vi "DSF.Engine.BuilderManager.Initialize Builders.vi"(7 "Framework Cache":refnum<class "DSF.Engine.Memory.Cache.Framework.lvclass">, 8 "error in (no error)":errorcluster, 10 "Builder Statuses":refnum<class "Status.Builder.lvclass">[](array[class]), 11 "Builder Manager in":refnum<class "DSF.Engine.BuilderManager.lvclass">) -> (0 "error out":errorcluster, 3 "Builder Manager out":refnum<class "DSF.Engine.BuilderManager.lvclass">)   [LabVIEW 2016, in "DSF.Engine.lvlib" / "DSF.Engine.BuilderManager.lvclass"]
uses:
  DSF.Engine.BuilderManager.lvclass
  Cache/DSF.Engine.Memory.Cache.Framework.lvclass
  Status/Status.Builder.lvclass
  DSF.Engine.BuilderManager.lvclass/DSF.Engine.BuilderManager.ctl
  Builder/DSF.Engine.Builder.lvclass
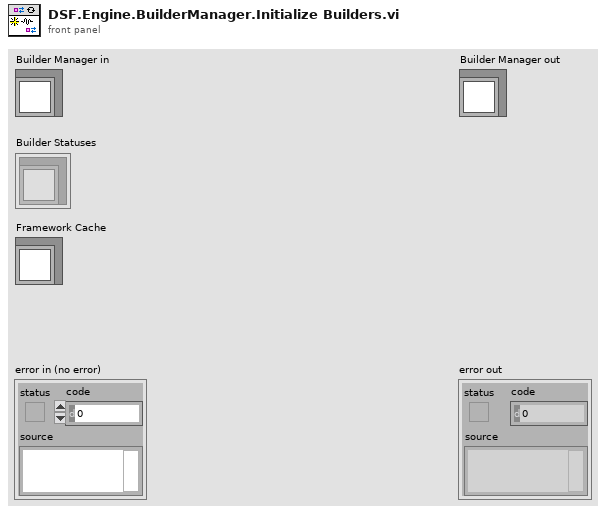
[diagram p1: front panel]
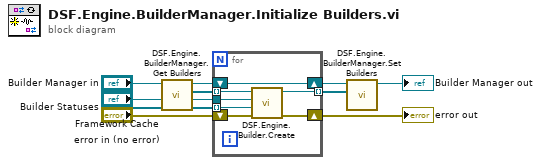
[diagram p0: block diagram]
diagram:
  n1 = call "DSF.Engine.BuilderManager.Get Builders.vi"("Builder Manager in"="Builder Manager in") -> ("Builders"=w8:refnum<class "DSF.Engine.Builder.lvclass">[], "Builder Manager out"=w7:refnum<class "DSF.Engine.BuilderManager.lvclass">)  [unwired: 9 in]
  n2 = for {
    tunnel: w8 -> [w16] mode=indexing
    shift-right: [w17] -> w6
    shift-left: w7 -> [w17]
    tunnel: [w15] -> w5 mode=indexing
    shift-right: [w14] -> w3
    shift-left: "error in (no error)" -> [w13]
    tunnel: "Builder Statuses" -> [w12] mode=indexing
    tunnel: "Framework Cache" -> [w11]
    n3 = call "DSF.Engine.Builder.Create.vi"("error in (no error)"=w13, "Builder Status"=w12, "Framework Cache"=w11, "Builder type"=w16) -> ("error out"=w14:errorcluster, "Builder"=w15:refnum<class "DSF.Engine.Builder.lvclass">)  [unwired: 6 in]
  }
  "error out" <- w3
  n4 = call "DSF.Engine.BuilderManager.Set Builders.vi"("Builders"=w5, "Builder Manager in"=w6) -> ("Builder Manager out"=→"Builder Manager out":refnum<class "DSF.Engine.BuilderManager.lvclass">)  [unwired: 9 in]
